vi "TAT_Com_PLC.vi"() -> ()   [LabVIEW 2017]
uses:
  <vilib>/NI/Modbus Library/API/Wrapper/Create TCP Master.vi
  Global/Global 1.vi
  <vilib>/NI/Modbus Library/API/Master/Modbus Master.lvclass
  <vilib>/NI/Modbus Library/API/Wrapper/API Main.lvlib
panel:
  out "Write to PLC":bool[](array[boolean])
  out "error out":errorcluster
  out "Array":i32[](array[numeric])
  out "PLC STATUS":bool
  in  "error in":errorcluster
  in  "stop":bool
  # "Ass & Leak"
  # "Station1--- Model selection 2012\ncycle start -- 2014\nLeak test OK ---2016\ncycle time---2018\nsensor1--2032\nsensor3---2034\n..sensor4---2048"
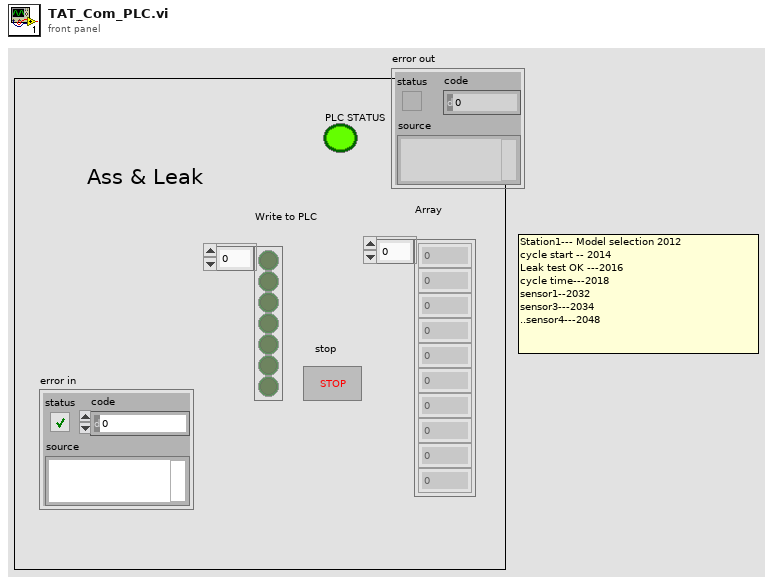
[diagram p1: front panel]
types:
  T1 = enum32{"invalid app kind", "Development System", "Run Time System", "Student Edition", "Embedded LabVIEW", "Evaluation", "Custom"}
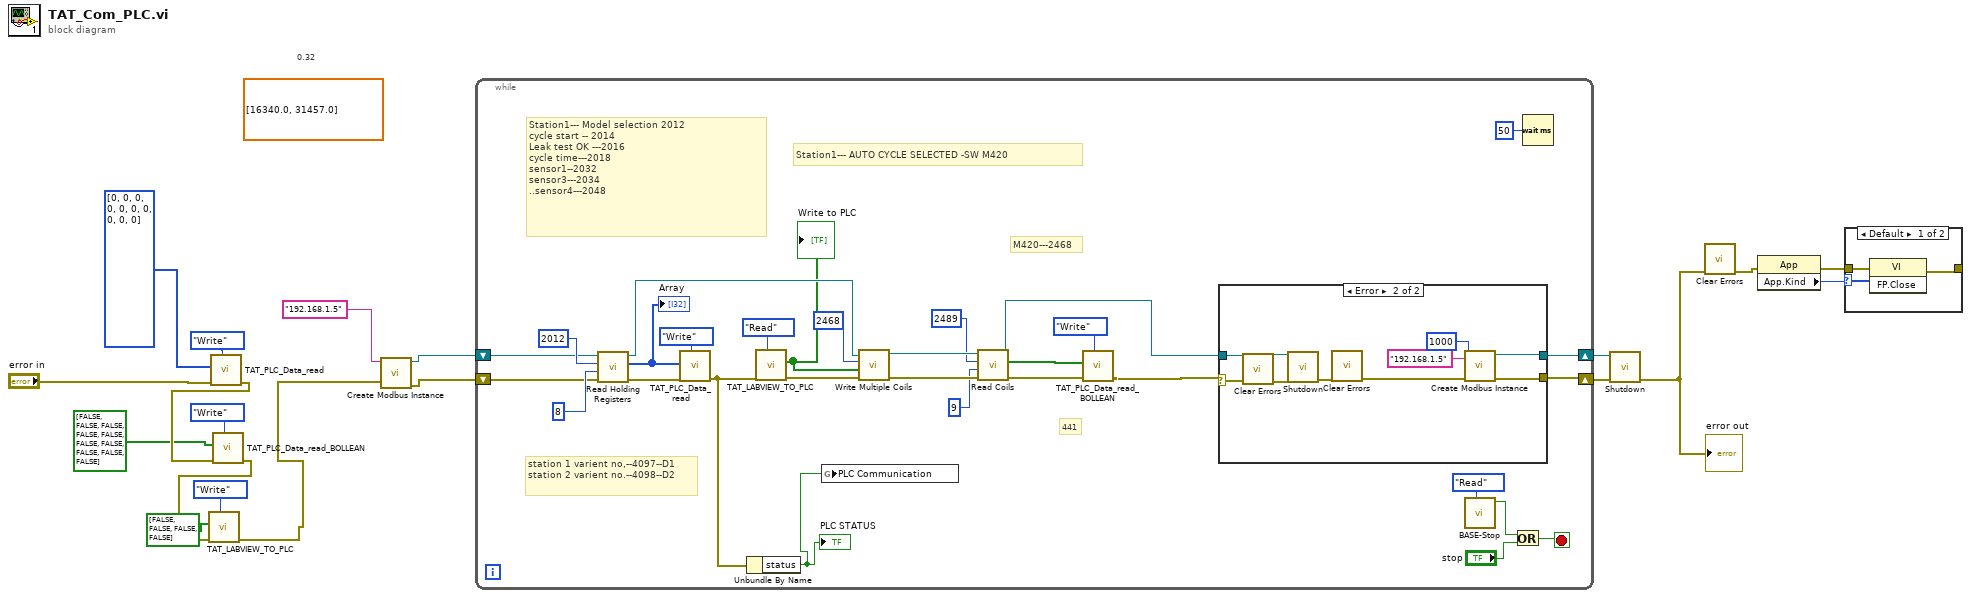
[diagram p0: block diagram]
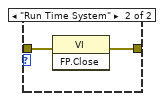
[diagram p3: hidden frame]
diagram:
  (unwired) dbl[] [16340.0, 31457.0] ("register values")
  # "0.32"
  n1 = call "TAT_PLC_Data_read.vi"("Enum"=enum16{"Read", "Write"}."Write", "error in (no error)"="error in", "Array"=i64[] [0, 0, 0, 0, 0, 0, 0, 0, 0, 0] ("Array 3")) -> ("error out"=w8:errorcluster)  [unwired: 7 in, 1 out]
  n2 = call "TAT_PLC_Data_read_BOLLEAN.vi"("Enum"=enum16{"Read", "Write"}."Write", "error in (no error)"=w8, "Array"=bool[] [FALSE, FALSE, FALSE, FALSE, FALSE, FALSE, FALSE, FALSE, FALSE, FALSE]) -> ("error out"=w4:errorcluster)  [unwired: 7 in, 1 out]
  n3 = call "TAT_LABVIEW_TO_PLC.vi"("Enum"=enum16{"Read", "Write"}."Write", "error in (no error)"=w4, "Array"=bool[] [FALSE, FALSE, FALSE, FALSE]) -> ("error out"=w5:errorcluster)  [unwired: 7 in, 1 out]
  n4 = call-poly <vilib>:"Create Modbus Instance.vi"("error in"=w5, "address"="192.168.1.5") -> ("error out"=w14:errorcluster, "TCP master instance"=w13:refnum<class "Modbus Master.lvclass">)  [unwired: 8 in]
  n5 = while {
    shift-right: [w47] -> w18
    shift-left: w13 -> [w42]
    shift-right: [w46] -> w17
    shift-left: w14 -> [w43]
    stop <- w48 stop-if-true
    # "441"
    # "M420---2468"
    # "Station1--- AUTO CYCLE SELECTED -SW M420"
    # "Station1--- Model selection 2012\ncycle start -- 2014\nLeak test OK ---2016\ncycle time---2018\nsensor1--2032\nsensor3---2034\n..sensor4---2048"
    # "station 1 varient no,--4097--D1\nstation 2 varient no.--4098--D2"
    n6 = call-dynamic "Read Holding Registers.vi"("error in"=w43, "number of inputs"=u16 8, "starting address"=u16 2012, "Modbus master in"=w42) -> ("error out"=w39:errorcluster, "register values"=w31:u16[], "Modbus master out"=w37:refnum<class "Modbus Master.lvclass">)  [unwired: 5 in]
    "Array" <- w31
    n7 = call "TAT_PLC_Data_read.vi"("Enum"=enum16{"Read", "Write"}."Write", "error in (no error)"=w39, "Array"=w31) -> ("error out"=w38:errorcluster)  [unwired: 7 in, 1 out]
    n8 = Unbundle By Name(w38) -> ("status"=w20:bool)
    "PLC STATUS" <- w20
    n9 = call "TAT_LABVIEW_TO_PLC.vi"("Enum"=enum16{"Read", "Write"}."Read", "error in (no error)"=w38) -> ("error out"=w35:errorcluster, "Array 2"=w30:bool[])  [unwired: 8 in]
    "Write to PLC" <- w30
    n10 = global write "Global 1.vi" "PLC Communication"(w20) -> ()
    n11 = call-dynamic "Write Multiple Coils.vi"("error in"=w35, "coils to write"=w30, "starting address"=u16 2468, "Modbus master in"=w37) -> ("error out"=w28:errorcluster, "Modbus master out"=w27:refnum<class "Modbus Master.lvclass">)  [unwired: 6 in]
    n12 = call-dynamic "Read Coils.vi"("error in"=w28, "number of inputs"=u16 9, "starting address"=u16 2489, "Modbus master in"=w27) -> ("error out"=w22:errorcluster, "coils"=w23:bool[], "Modbus master out"=w26:refnum<class "Modbus Master.lvclass">)  [unwired: 5 in]
    n13 = call "TAT_PLC_Data_read_BOLLEAN.vi"("Enum"=enum16{"Read", "Write"}."Write", "error in (no error)"=w22, "Array"=w23) -> ("error out"=w21:errorcluster)  [unwired: 7 in, 1 out]
    n14 = case shown="Error" w21 {
      selector: w21 -> [w50 w60]
      tunnel: w26 -> [w51 w58]
      tunnel: [w51 w54] -> w47
      tunnel: [w50 w53] -> w46
      frame No Error {
      }
      frame Error {
        n15 = call <vilib>:"Clear Errors.vi"("error in (no error)"=w60) -> ("error out"=w59:errorcluster)  [unwired: 5 in, 1 out]
        n16 = call-dynamic "Shutdown.vi"("error in"=w59, "Modbus master in"=w58) -> ("error out"=w57:errorcluster)  [unwired: 9 in]
        n17 = call <vilib>:"Clear Errors.vi"("error in (no error)"=w57) -> ("error out"=w55:errorcluster)  [unwired: 5 in, 1 out]
        n18 = call-poly <vilib>:"Create Modbus Instance.vi"("error in"=w55, "connect timeout ms"=1000, "address"="192.168.1.5") -> ("error out"=w53:errorcluster, "TCP master instance"=w54:refnum<class "Modbus Master.lvclass">)  [unwired: 7 in]
      }
    }
    n19 = call "BASE-Stop.vi"("Enum"=enum16{"Read", "Write"}."Read") -> ("Stop"=w32:bool)  [unwired: 10 in]
    n20 = Or(x=w32, y="stop") -> (x .or. y?=w48:bool)
    n21 = Wait (ms)(milliseconds to wait=u32 50) -> ()  [unwired: 1 out]
  }
  n22 = call-dynamic "Shutdown.vi"("error in"=w17, "Modbus master in"=w18) -> ("error out"=w2:errorcluster)  [unwired: 9 in]
  "error out" <- w2
  n23 = call <vilib>:"Clear Errors.vi"("error in (no error)"=w2) -> ("error out"=w1:errorcluster)  [unwired: 5 in, 1 out]
  n24 = property class="App"(error in=w1) -> (error out=w15:errorcluster, "App.Kind"=w16:T1)  [unwired: 1 in, 1 out]
  n25 = case shown="Default" w16 {
    tunnel: w15 -> [w62 w64]
    tunnel: [w61 w63] -> _
    frame Default {
      n26 = invoke class="VI" method="FP.Close"(error in=w62) -> (error out=w61:errorcluster)  [unwired: 2 in, 2 out]
    }
    frame "Run Time System" {
      n27 = invoke class="VI" method="FP.Close"(error in=w64) -> (error out=w63:errorcluster)  [unwired: 2 in, 2 out]
    }
  }
